vi "Set H2H Flag Based on H2H Flag Array.vi"(9 "This Row":i32[](array[numeric]), 10 "H2H Flag Array":bool[][](array[boolean]), 11 "Flag Array":bool[][](array[boolean])) -> (3 "Flag Array Out":bool[][](array[boolean]))   [LabVIEW 2013]
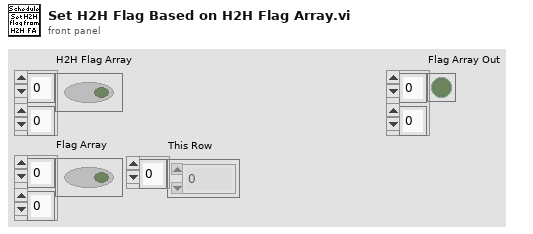
[diagram p1: front panel]
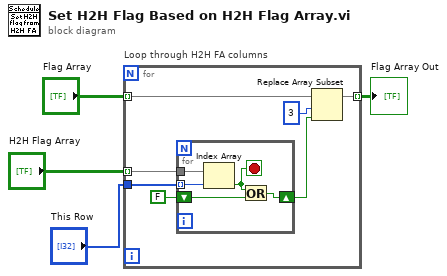
[diagram p0: block diagram]
diagram:
  n1 = for "Loop through H2H FA columns" {
    tunnel: "H2H Flag Array" -> [w9] mode=indexing
    tunnel: "Flag Array" -> [w8] mode=indexing
    tunnel: "This Row" -> [w11]
    tunnel: [w5] -> w1 mode=indexing
    n2 = for {
      tunnel: w11 -> [w15] mode=indexing
      shift-right: [w14] -> w6
      shift-left: FALSE -> [w13]
      tunnel: w9 -> [w16]
      stop <- w12 stop-if-true
      n3 = Index Array(array=w16, index=w15) -> (element=w12:bool)
      n4 = Or(x=w12, y=w13) -> (x .or. y?=w14:bool)
    }
    n5 = Replace Array Subset(array=w8, new element=w6, index=3) -> (w5:bool[])
  }
  "Flag Array Out" <- w1
